vi "prova.vi"   [LabVIEW 2015]
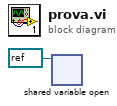
[diagram p0: block diagram]
diagram:
  n1 = shared-variable-open(refnum<k21> refnum ("shared variable refnum in")) -> ()  [unwired: 5 in, 2 out]
